vi "报警页面.vi"() -> ()   [LabVIEW 2015]
panel:
  out "时间":string
  out "日期":string
  in  "报警列表翻页至顶":bool
  in  "报警列表向上翻页":bool
  in  "报警列表向下翻页":bool
  in  "报警声音消音":bool
  in  "确认所选报警":bool
  in  "确认当前画面所有报警":bool
  in  "多列列表框":i32(listbox)
  # "报警页面"
  # "确认任务"
  # "报警画面任务"
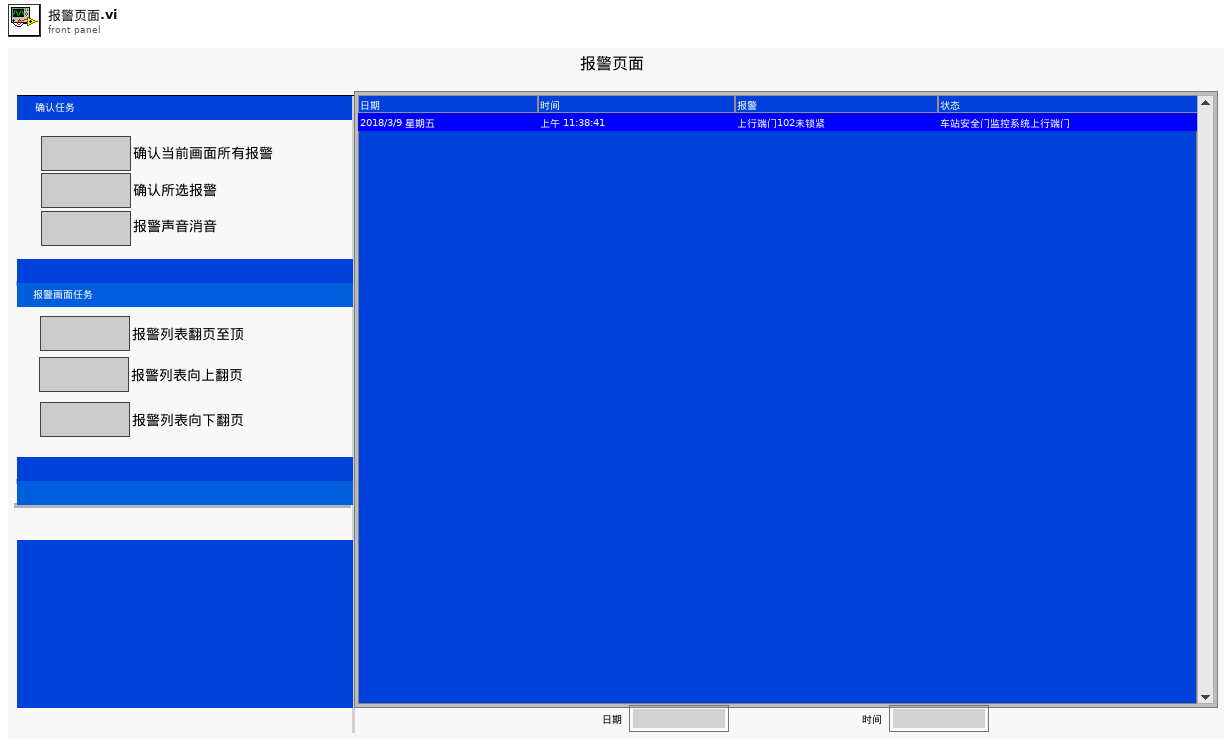
[diagram p1: front panel]
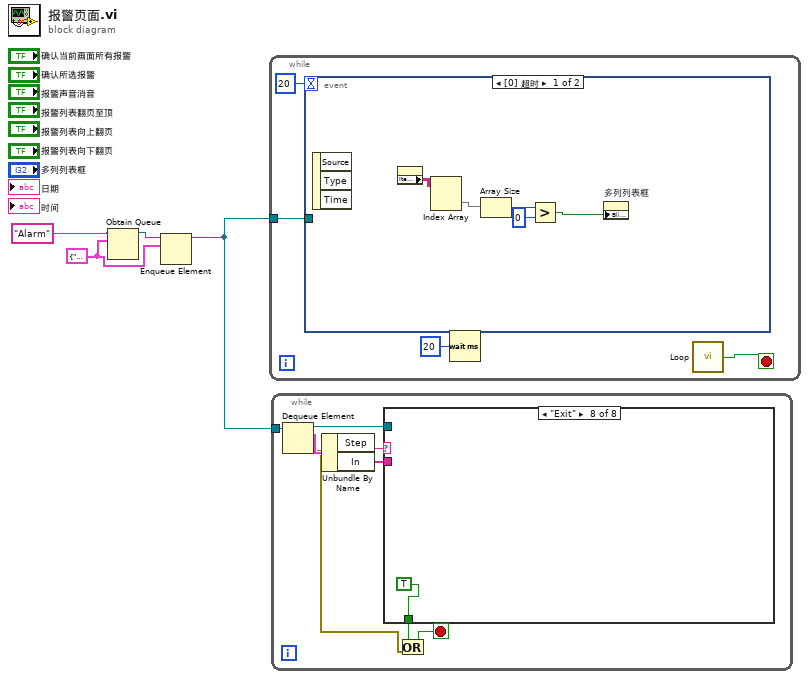
[diagram p0: block diagram]
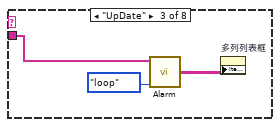
[diagram p4: hidden frame]
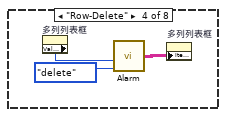
[diagram p5: hidden frame]
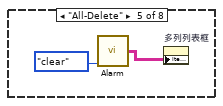
[diagram p6: hidden frame]
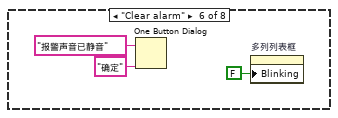
[diagram p7: hidden frame]
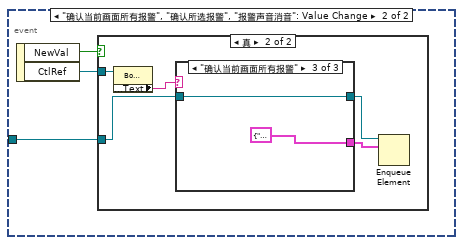
[diagram p9: hidden frame]
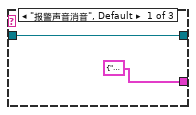
[diagram p11: hidden frame]
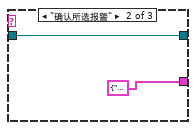
[diagram p12: hidden frame]
diagram:
  w1 = cluster{"Step\n":string, "In":string[]} {"Step\n"="All-Delete", "In"=[]}
  n1 = Obtain Queue(name (unnamed)="Alarm" ("名称（未命名）"), element data type=w1) -> (queue out=w3:refnum<queue>)  [unwired: 3 in, 2 out]
  n2 = Enqueue Element(queue=w3, element=w1) -> (queue out=w2:refnum<queue>)  [unwired: 2 in, 2 out]
  n3 = while {
    tunnel: w2 -> [w7]
    stop <- w8 stop-if-true
    n4 = event shown="[0] 超时" {
      selector: _ -> [_ _]
      dyn-events: _ -> [_ _]
      timeout: 20 -> [_ _]
      tunnel: w7 -> [_ w14]
      event Timeout {
        n5 = event-data() -> ()  [unwired: 1 in, 3 out]
        n6 = property on="多列列表框" class="MCListbox (严格)"() -> ("ItemNames"=w13:string[][])  [unwired: 2 in, 2 out]
        n7 = Index Array(array=w13) -> (element=w12:string[])  [unwired: 2 in]
        n8 = Array Size(array=w12) -> (size(s)=w11:i32)
        n9 = Greater?(x=w11, y=0) -> (0:w9:bool)
        n10 = property on="多列列表框" class="MCListbox (严格)"("Blinking"=w9) -> ()  [unwired: 2 in, 2 out]
      }
      event "确认当前画面所有报警", "确认所选报警", "报警声音消音": Value Change {
        n11 = event-data() -> ("NewVal"=w16:bool, "CtlRef"=w15:refnum<vi>)  [unwired: 1 in]
        n12 = case shown="真" w16 {
          tunnel: w15 -> [_ w21]
          tunnel: w14 -> [_ w19]
          frame False {
          }
          frame True {
            n13 = property class="Bool (严格)"(reference=w21) -> ("Label.Text"=w20:string)  [unwired: 1 in, 2 out]
            n14 = case shown="\"确认当前画面所有报警\"" w20 {
              tunnel: w19 -> [w22 w25 w27]
              tunnel: [w22 w25 w27] -> w18
              tunnel: [cluster{"Step\n":string, "In":string[]} {"Step\n"="Clear alarm", "In"=[]} cluster{"Step\n":string, "In":string[]} {"Step\n"="Row-Delete", "In"=[]} cluster{"Step\n":string, "In":string[]} {"Step\n"="All-Delete", "In"=[]}] -> w17
              frame "报警声音消音", Default {
              }
              frame "确认所选报警" {
              }
              frame "确认当前画面所有报警" {
              }
            }
            n15 = Enqueue Element(queue=w18, element=w17) -> ()  [unwired: 2 in, 3 out]
          }
        }
      }
    }
    n16 = Wait (ms)(milliseconds to wait=u32 20 ("等待时间（毫秒）")) -> ()  [unwired: 1 out]
    n17 = call "Loop.vi"() -> ("Loop Out"=w8:bool)  [unwired: 5 in]
  }
  n18 = while {
    tunnel: w2 -> [w35]
    stop <- w29 stop-if-true
    n19 = Dequeue Element(queue=w35) -> (queue out=w34:refnum<queue>, element=w33:cluster{"Step\n":string, "In":string[]}, error out=w31:errorcluster)  [unwired: 2 in, 1 out]
    n20 = Unbundle By Name(w33) -> ("Step"=w32:string, "In"=w28:string[])
    n21 = case shown="\"Exit\"" w32 {
      tunnel: w34 -> [_ _ _ _ _ _ _ _]
      tunnel: [_ _ _ _ _ _ _ TRUE] -> w30
      tunnel: w28 -> [_ _ w37 _ _ _ _ _]
      frame "假", Default {
      }
      frame "Init" {
      }
      frame "UpDate" {
        n22 = call "Alarm.vi"("Lable"=enum16{"UpDate", "loop", "delete", "clear"}."loop", "In"=w37) -> ("Out"=w36:string[][])  [unwired: 4 in]
        n23 = property on="多列列表框" class="MCListbox (严格)"("ItemNames"=w36) -> ()  [unwired: 2 in, 2 out]
      }
      frame "Row-Delete" {
        n24 = property on="多列列表框" class="MCListbox (严格)"() -> ("Value"=w40:i32)  [unwired: 2 in, 2 out]
        n25 = call "Alarm.vi"("Lable"=enum16{"UpDate", "loop", "delete", "clear"}."delete", "Delete Row"=w40) -> ("Out"=w39:string[][])  [unwired: 4 in]
        n26 = property on="多列列表框" class="MCListbox (严格)"("ItemNames"=w39) -> ()  [unwired: 2 in, 2 out]
      }
      frame "All-Delete" {
        n27 = call "Alarm.vi"("Lable"=enum16{"UpDate", "loop", "delete", "clear"}."clear") -> ("Out"=w42:string[][])  [unwired: 5 in]
        n28 = property on="多列列表框" class="MCListbox (严格)"("ItemNames"=w42) -> ()  [unwired: 2 in, 2 out]
      }
      frame "Clear alarm" {
        n29 = One Button Dialog(message="报警声音已静音" ("消息"), button name ("OK")="确定" ("按钮名称（“确定”）")) -> ()  [unwired: 1 out]
        n30 = property on="多列列表框" class="MCListbox (严格)"("Blinking"=FALSE ("闪烁")) -> ()  [unwired: 2 in, 2 out]
      }
      frame "Stick" {
      }
      frame "Exit" {
      }
    }
    n31 = Or(x=w30, y=w31) -> (x .or. y?=w29:bool)
  }
